vi "exit_main.vi"(0 "Dieses VI":refnum<vi>, 1 "deutsch?":bool, 2 "balance":refnum<vi>, 4 "volume":refnum<vi>, 5 "configPfad":refnum<vi>, 6 "notifyicon_reference":refnum<vi>, 7 "verdeckung":refnum<vi>) -> ()   [LabVIEW 2012]
uses:
  musicplayer_glo.vi
  player_glo.vi
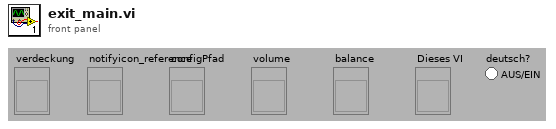
[diagram p1: front panel]
types:
  T1 = enum16{"Left Button", "Center Button", "Right Button", "Window Close"}
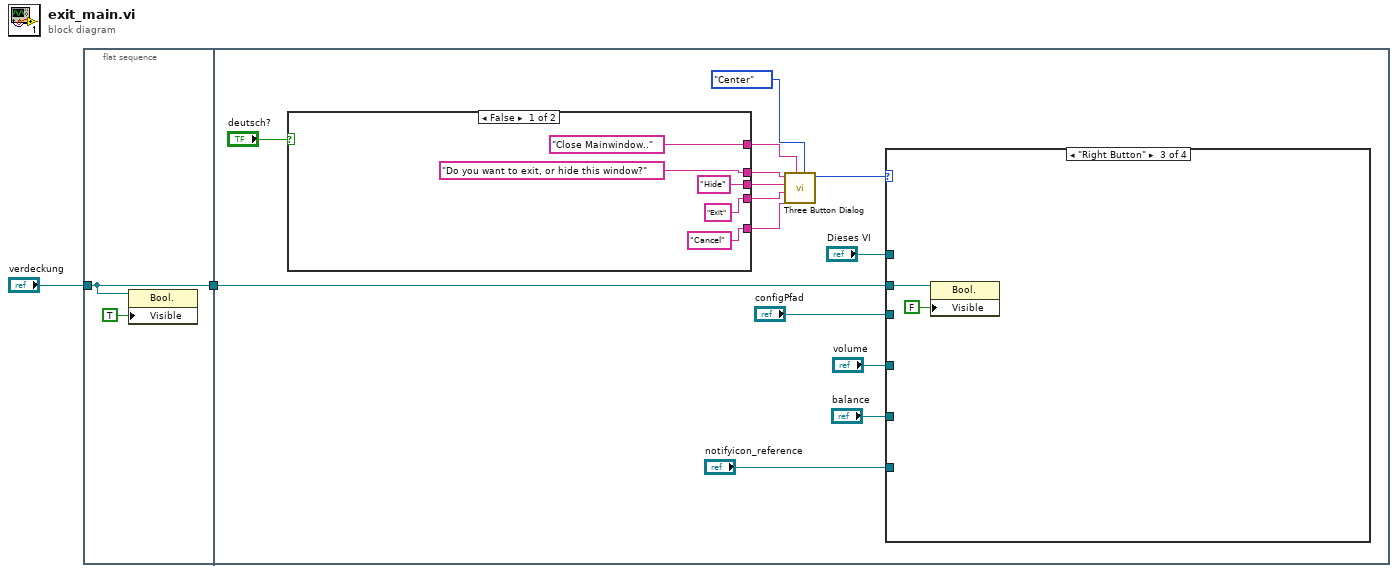
[diagram p0: block diagram]
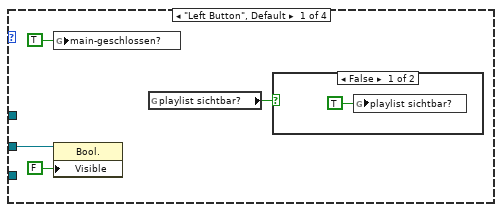
[diagram p2: hidden frame]
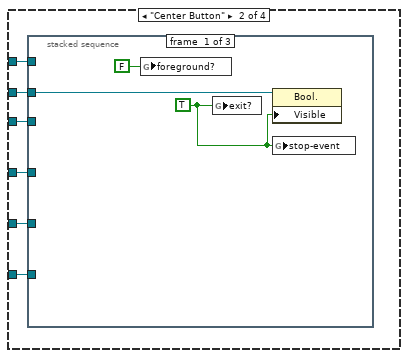
[diagram p4: hidden frame]
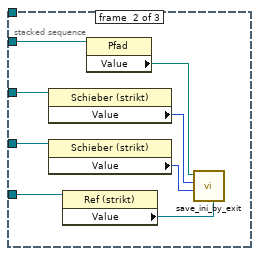
[diagram p5: hidden frame]
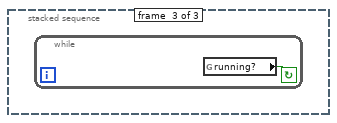
[diagram p6: hidden frame]
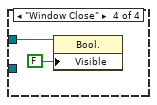
[diagram p7: hidden frame]
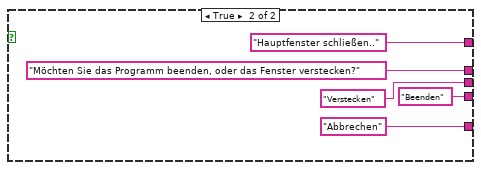
[diagram p8: hidden frame]
diagram:
  n1 = flat-sequence {
    tunnel: [w4] -> w2
    tunnel: "verdeckung" -> [w4]
    tunnel: w2 -> [w5]
    frame #0 {
      n2 = property class="Bool."(reference=w4, "Visible"=TRUE ("Sichtbar")) -> ()  [unwired: 1 in, 2 out]
    }
    frame #1 {
      n3 = case shown="False" "deutsch?" {
        tunnel: ["Close Mainwindow.." "Hauptfenster schließen.."] -> w18
        tunnel: ["Do you want to exit, or hide this window?" "Möchten Sie das Programm beenden, oder das Fenster verstecken?"] -> w17
        tunnel: ["Hide" "Verstecken"] -> w16
        tunnel: ["Exit" "Beenden"] -> w15
        tunnel: ["Cancel" "Abbrechen"] -> w14
        frame False {
        }
        frame True {
        }
      }
      n4 = call <vilib>:"Three Button Dialog.vi"("Justify Message (Left)"=enum16{"Left", "Center", "Right"}."Center", "Window Title (\"\")"=w18, "Right Button Text (\"Cancel\")"=w14, "Center Button Text (\"No\")"=w15, "Left Button Text (\"Yes\")"=w16, "message"=w17) -> ("Which Button?"=w12:T1)  [unwired: 5 in]
      n5 = case shown="\"Right Button\"" w12 {
        tunnel: "Dieses VI" -> [_ w29 _ _]
        tunnel: w5 -> [w19 w28 w42 w45]
        tunnel: "notifyicon_reference" -> [_ w27 _ _]
        tunnel: "configPfad" -> [_ w26 _ _]
        tunnel: "volume" -> [_ w25 _ _]
        tunnel: "balance" -> [_ w24 _ _]
        frame "Left Button", Default {
          n6 = global write "musicplayer_glo.vi" "main-geschlossen?"(TRUE) -> ()
          n7 = property class="Bool."(reference=w19, "Visible"=FALSE ("Sichtbar")) -> ()  [unwired: 1 in, 2 out]
          n8 = global read "musicplayer_glo.vi" "playlist sichtbar?"() -> (w21:bool)
          n9 = case shown="False" w21 {
            frame False {
              n10 = global write "musicplayer_glo.vi" "playlist sichtbar?"(TRUE) -> ()
            }
            frame True {
            }
          }
        }
        frame "Center Button" {
          n11 = stacked-sequence {
            tunnel: w29 -> [_ _ _]
            tunnel: w28 -> [w30 _ _]
            tunnel: w27 -> [_ w36 _]
            tunnel: w26 -> [_ w35 _]
            tunnel: w25 -> [_ w34 _]
            tunnel: w24 -> [_ w33 _]
            frame #0 {
              w32 = TRUE ("stop-event")
              n12 = global write "musicplayer_glo.vi" "foreground?"(FALSE ("foreground?")) -> ()
              n13 = global write "musicplayer_glo.vi" "exit?"(w32) -> ()
              n14 = property on="Eigenschaftsknoten" class="Bool."(reference=w30, "Visible"=w32) -> ()  [unwired: 1 in, 2 out]
              n15 = global write "musicplayer_glo.vi" "stop-event"(w32) -> ()
            }
            frame #1 {
              n16 = property class="Schieber (strikt)"(reference=w34) -> ("Value"=w38:i64)  [unwired: 1 in, 2 out]
              n17 = property class="Schieber (strikt)"(reference=w33) -> ("Value"=w37:i8)  [unwired: 1 in, 2 out]
              n18 = property class="Ref (strikt)"(reference=w36) -> ("Value"=w40:refnum<k24>)  [unwired: 1 in, 2 out]
              n19 = property class="Pfad"(reference=w35) -> ("Value"=w39:path)  [unwired: 1 in, 2 out]
              n20 = call "save_ini_by_exit.vi"("NotifyIcon reference"=w40, "balance"=w37, "volume"=w38, "einstellungspfad"=w39) -> ()  [unwired: 8 in]
            }
            frame #2 {
              n21 = while {
                stop <- w41 continue-if-true
                n22 = global read "player_glo.vi" "running?"() -> (w41:bool)
              }
            }
          }
        }
        frame "Right Button" {
          n23 = property class="Bool."(reference=w42, "Visible"=FALSE ("Sichtbar")) -> ()  [unwired: 1 in, 2 out]
        }
        frame "Window Close" {
          n24 = property class="Bool."(reference=w45, "Visible"=FALSE ("Sichtbar")) -> ()  [unwired: 1 in, 2 out]
        }
      }
    }
  }
